vi "colocviu.vi"() -> ()   [LabVIEW 2011]
panel:
  out "Thermometer":dbl(slide) scale=0.0..10.0
  out "Raportul Nr.1 / Nr. 2":dbl
  out "Diferenta Nr.1 - Nr2":dbl
  in  "stop":bool
  out "Meter":dbl(knob) scale=-10.0..10.0
  in  "Nr. 1":dbl(slide) scale=0.0..10.0
  in  "Nr. 2":dbl(slide) scale=0.0..10.0
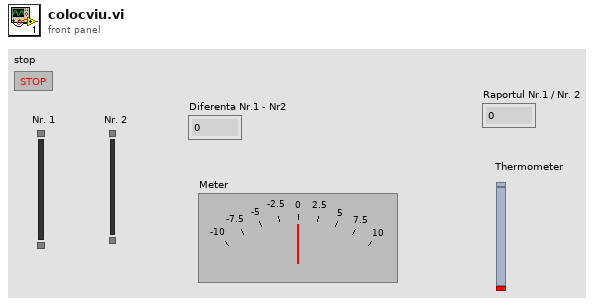
[diagram p1: front panel]
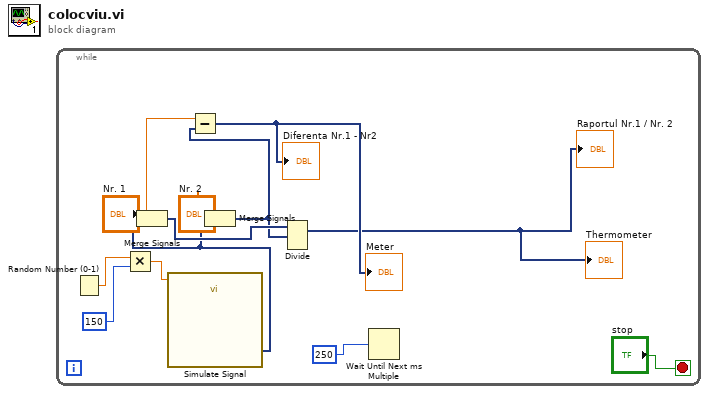
[diagram p0: block diagram]
diagram:
  n1 = while {
    stop <- "stop" stop-if-true
    n2 = Random Number (0-1)() -> (number: 0 to 1=w6:dbl)
    n3 = Multiply(x=w6, y=150) -> (x*y=w4:dbl)
    n4 = call "Simulate Signal"("Offset"=w4) -> ("Sine"=w1:dynamicdata)  [unwired: 13 in, 1 out]
    n5 = Merge Signals("Nr. 1", w1) -> (w3:dynamicdata)
    n6 = Merge Signals("Nr. 2", w1) -> (w2:dynamicdata)
    n7 = Subtract(x="Nr. 1", y=w2) -> (x-y=→"Meter" →"Diferenta Nr.1 - Nr2":dynamicdata)
    n8 = Divide(1:w2, 2:w3) -> (0:→"Raportul Nr.1 / Nr. 2" →"Thermometer":dynamicdata)  [unwired: 1 in, 1 out]
    n9 = Wait Until Next ms Multiple(millisecond multiple=250) -> ()  [unwired: 1 out]
  }
